vi "Set Via App.vi"(8 "error in (no error)":errorcluster, 10 "ViaApp":refnum<class "ViaApp.lvclass">, 11 "GWebAppArrayPanel in":refnum<class "GWebAppArrayPanel.lvclass">) -> (0 "error out":errorcluster, 3 "GWebAppArrayPanel out":refnum<class "GWebAppArrayPanel.lvclass">)   [LabVIEW 2020, in "PicoG-App.lvlib" / "GWebAppArrayPanel.lvclass"]
uses:
  GWebAppArrayPanel.lvclass
  ViaApp/ViaApp.lvclass
  GWebAppArrayPanel.lvclass/GWebAppArrayPanel.ctl
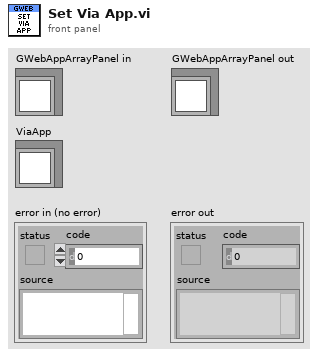
[diagram p1: front panel]
types:
  T1 = typedef "PicoG-App.lvlib/GWebAppArrayPanel.lvclass/Ref Data.ctl" = cluster{"App":refnum<class "ViaApp.lvclass">}
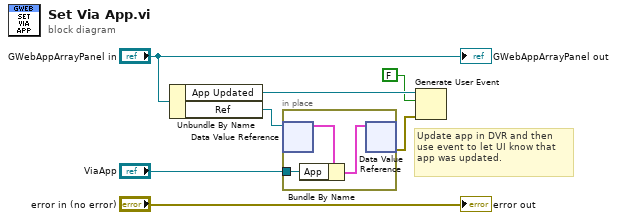
[diagram p0: block diagram]
diagram:
  # "Update app in DVR and then use event to let UI know that app was updated."
  n1 = Unbundle By Name("GWebAppArrayPanel in") -> ("App Updated"=w3:refnum<user-event>, "Ref"=w6:refnum<data-value>)
  n2 = in-place {
    in-place-border: "ViaApp" -> [w8]
    n3 = in-place-dvr #1(w6) -> (w10:T1)  [unwired: 1 out]
    n4 = Bundle By Name(cluster=w10, "App"=w8) -> (w9:T1)
    n5 = in-place-dvr #1(w9) -> (w2:errorcluster)  [unwired: 1 out]
  }
  n6 = Generate User Event(user event=w3, event data cluster=FALSE ("event data"), error in=w2) -> ()  [unwired: 1 in, 2 out]
  "error out" <- "error in (no error)"
  "GWebAppArrayPanel out" <- "GWebAppArrayPanel in"
